vi "TEST_Shadow.vi"   [LabVIEW 2021, in "UIShadow.lvlib"]
uses:
  UIShadow.lvlib
  Shadow.lvclass
types:
  T1 = enum32{"Invalid", "Standard", "Closed", "Hidden", "Minimized", "Maximized"}
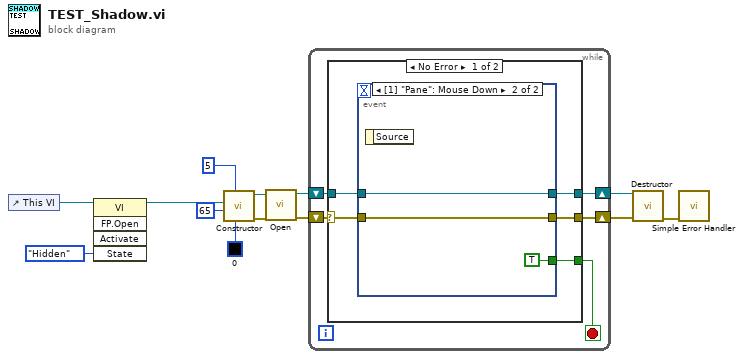
[diagram p0: block diagram]
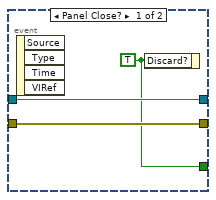
[diagram p2: hidden frame]
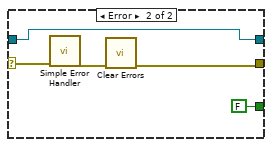
[diagram p3: hidden frame]
diagram:
  n1 = control-ref of="This VI"() -> (w9:refnum<vi>)
  n2 = invoke class="VI" method="FP.Open"(reference=w9, "State"=T1."Hidden") -> (reference out=w7:refnum<vi>)  [unwired: 3 in, 4 out]
  n3 = call "Constructor.vi"("ShadowColor"=u32 0, "Offset"=i16 5, "Transparancy"=65, "VI Refnum"=w7) -> ("error out"=w12:errorcluster, "Shadow out"=w13:refnum<class "Shadow.lvclass">)  [unwired: 6 in]
  n4 = call "Open.vi"("error in (no error)"=w12, "Shadow in"=w13) -> ("error out"=w11:errorcluster, "Shadow out"=w10:refnum<class "Shadow.lvclass">)  [unwired: 8 in]
  n5 = while {
    shift-right: [w15] -> w2
    shift-left: w10 -> [w18]
    shift-right: [w16] -> w1
    shift-left: w11 -> [w17]
    stop <- w14 stop-if-true
    n6 = case shown="No Error" w17 {
      selector: w17 -> [w22 w34]
      tunnel: w18 -> [w23 w32]
      tunnel: [w21 w31] -> w16
      tunnel: [w20 w32] -> w15
      tunnel: [w19 FALSE ("Discard?")] -> w14
      frame No Error {
        n7 = event shown="[1] \"Pane\": Mouse Down" {
          selector: _ -> [_ _]
          dyn-events: _ -> [_ _]
          timeout: _ -> [_ _]
          tunnel: w23 -> [w25 w28]
          tunnel: [w26 w27] -> w21
          tunnel: w22 -> [w26 w27]
          tunnel: [w25 w28] -> w20
          tunnel: [w24 TRUE ("Discard?")] -> w19
          event Panel Close? {
            w24 = TRUE ("Discard?")
            n8 = event-data() -> ()  [unwired: 1 in, 4 out]
            n9 = event-data("Discard?"=w24) -> ()  [unwired: 1 in, 1 out]
          }
          event Mouse Down {
            n10 = event-data() -> ()  [unwired: 1 in, 1 out]
          }
        }
      }
      frame Error {
        n11 = call <vilib>:"Simple Error Handler.vi"("error in (no error)"=w34) -> ("error out"=w33:errorcluster)  [unwired: 4 in, 4 out]
        n12 = call <vilib>:"Clear Errors.vi"("error in (no error)"=w33) -> ("error out"=w31:errorcluster)  [unwired: 5 in, 1 out]
      }
    }
  }
  n13 = call "Destructor.vi"("error in (no error)"=w1, "Shadow in"=w2) -> ("error out"=w8:errorcluster)  [unwired: 9 in]
  n14 = call <vilib>:"Simple Error Handler.vi"("error in (no error)"=w8) -> ()  [unwired: 4 in, 5 out]
